vi "ID组合.vi"(8 "SA(4)":i32 format="%x", 9 "PS(3)":i32 format="%x", 10 "PF(2)":i32 format="%x", 11 "PDU(1)":i32 format="%x") -> (3 "ID":i32 format="%x")   [LabVIEW 2013]
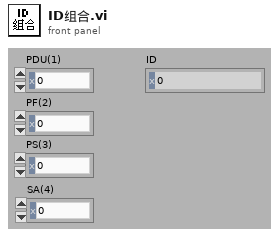
[diagram p1: front panel]
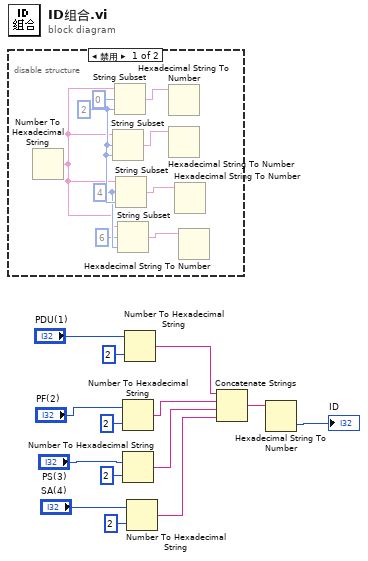
[diagram p0: block diagram]
diagram:
  n1 = disable-structure shown="禁用" {
    frame Disabled {
      w21 = 4 ("偏移量(0)")
      w22 = 2 ("长度（剩余）")
      n2 = Number To Hexadecimal String() -> (0:w19:string)  [unwired: 1 in, 1 out]
      n3 = String Subset(string=w19, offset (0)=w22, length (rest)=w22) -> (substring=w17:string)
      n4 = String Subset(string=w19, offset (0)=0 ("偏移量(0)"), length (rest)=w22) -> (substring=w18:string)
      n5 = String Subset(string=w19, offset (0)=w21, length (rest)=w22) -> (substring=w16:string)
      n6 = String Subset(string=w19, offset (0)=6 ("偏移量(0)"), length (rest)=w21) -> (substring=w15:string)
      n7 = Hexadecimal String To Number(string=w18) -> ()  [unwired: 4 out]
      n8 = Hexadecimal String To Number(string=w17) -> ()  [unwired: 4 out]
      n9 = Hexadecimal String To Number(string=w16) -> ()  [unwired: 4 out]
      n10 = Hexadecimal String To Number(string=w15) -> ()  [unwired: 4 out]
    }
    frame Enabled {
    }
  }
  n11 = Number To Hexadecimal String(1:i16 2 ("宽度(-)"), 2:"PF(2)") -> (0:w5:string)
  n12 = Number To Hexadecimal String(1:i16 2 ("宽度(-)"), 2:"PS(3)") -> (0:w4:string)
  n13 = Number To Hexadecimal String(1:i16 2 ("宽度(-)"), 2:"PDU(1)") -> (0:w6:string)
  n14 = Number To Hexadecimal String(1:i16 2 ("宽度(-)"), 2:"SA(4)") -> (0:w3:string)
  n15 = Concatenate Strings(w6, w5, w4, w3) -> (w2:string)
  n16 = Hexadecimal String To Number(string=w2) -> (number=→"ID":u32)  [unwired: 3 out]
